vi "test Verify with Regex Scrubber with Numbered Replacement.vi"(8 "error in":errorcluster, 11 "Testing Approval Tests in":refnum<class "VITester Extension Tests.lvclass">) -> (0 "error out":errorcluster, 3 "Testing Approval Tests out":refnum<class "VITester Extension Tests.lvclass">)   [LabVIEW 2020, in "VITester Extension Tests.lvclass"]
uses:
  VITester Extension Tests.lvclass
  Source/Approval Tests/Options.ctl
  Source/Approval Tests/Reporter/Reporter.lvclass
  Source/Approval Tests/Namer/Namer.lvclass
  Source/Approval Tests/Scrubber/Scrubber.lvclass
  Source/Approval Tests/Regex Scrubber With Numbered Replacements/Regex Scrubber with Numbered Replacement.lvclass
  C:/Users/SAS/Desktop/ApprovalTests.LabVIEW/Source/Approval Tests/Scrubber/Scrubber.lvclass
  Source/Approval Tests/Regex Scrubber With Numbered Replacements/Regex Scrubber with Numbered Replacement.lvclass/Regex Scrubber with Numbered Replacement.ctl
  c85dbac9-9df1-4385-95da-0d0c429ccc49.vi
  Source/Approval Tests/Regex Scrubber With Numbered Replacements/Write Regex.vi
  Source/Approval Tests/Regex Scrubber With Numbered Replacements/Write Prefix.vi
  c85dbac9-9df1-4385-95da-0d0c429ccc49.vi/ef028380-787c-4fa5-86c8-b0b7860ce2dc.vi
  c85dbac9-9df1-4385-95da-0d0c429ccc49.vi/ef028380-787c-4fa5-86c8-b0b7860ce2dc.vi/93c5622b-9fb7-41e0-8c76-3fde37e94e34.vi
  Source/Approval Tests/Replace with Caller if Empty.vi
  Source/Approval Tests/conv EOL.vi
  <vilib>/Utility/libraryn.llb/Check if File or Folder Exists.vi
  VITester Extension Tests.lvclass/VITester Extension Tests.ctl
  Source/Approval Tests/Approval Tests.lvlib
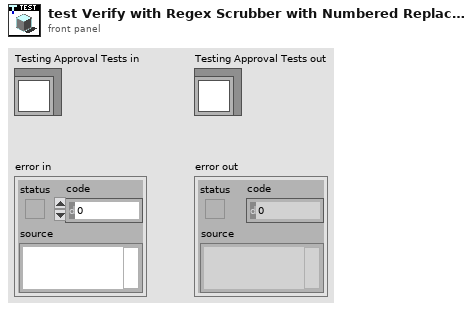
[diagram p1: front panel]
types:
  T1 = typedef "Approval Tests.lvlib/Options.ctl" = cluster{"Reporter":refnum<class "Reporter.lvclass">, "Extension(txt)":string, "Namer":refnum<class "Namer.lvclass">, "Scrubber":refnum<class "Scrubber.lvclass">, "Test Label":string}
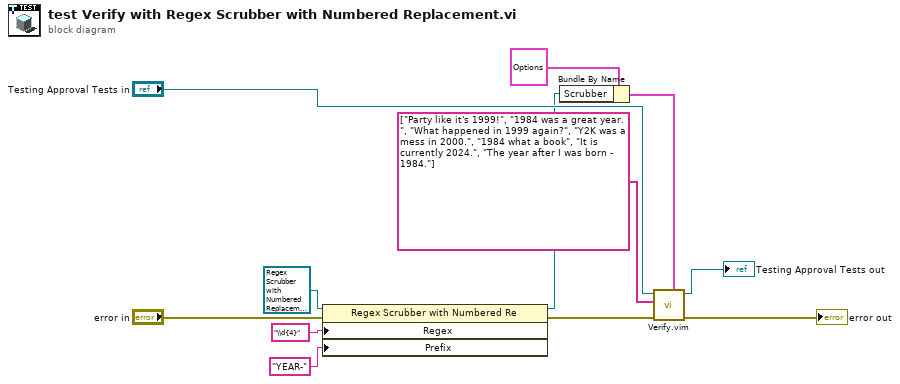
[diagram p0: block diagram]
diagram:
  n1 = property on="Property Node" class="Regex Scrubber with Numbered Re"(reference=refnum<class "Regex Scrubber with Numbered Replacement.lvclass"> refnum ("Approval Tests.lvlib:Regex Scrubber with Numbered Replacement.lvclass"), error in="error in", "Regex"="\\d{4}", "Prefix"="YEAR-" ("Replacement")) -> (reference out=w7:refnum<class "Regex Scrubber with Numbered Replacement.lvclass">, error out=w10:errorcluster)
  n2 = Bundle By Name(cluster=T1 {"Reporter"=refnum, "Extension(txt)"="", "Namer"=refnum, "Scrubber"=refnum, "Test Label"=""} ("Options"), "Scrubber"=w7) -> (w3:T1)
  n3 = call "Verify.vim"("Options"=w3, "error in"=w10, "Test Data"=string[] ["Party like it's 1999!", "1984 was a great year.", "What happened in 1999 again?", "Y2K was a mess in 2000.", "1984 what a book", "It is currently 2024.", "The year after I was born - 1984."], "TestCase"="Testing Approval Tests in") -> ("error out"=→"error out":errorcluster, "TestCase"=→"Testing Approval Tests out":refnum<class "VITester Extension Tests.lvclass">)  [unwired: 6 in]
